vi "Verify Message Type.vi"(8 "error in":errorcluster, 11 "message type in":string) -> (0 "error out":errorcluster, 3 "message type out":T1, 4 "expected RT direction":string, 6 "number of expected addresses":i32)   [LabVIEW 2020, in "MIL-STD 1553 Import.lvlib"]
uses:
  MIL-STD 1553 Import.lvlib
  Shared/Message Type.ctl
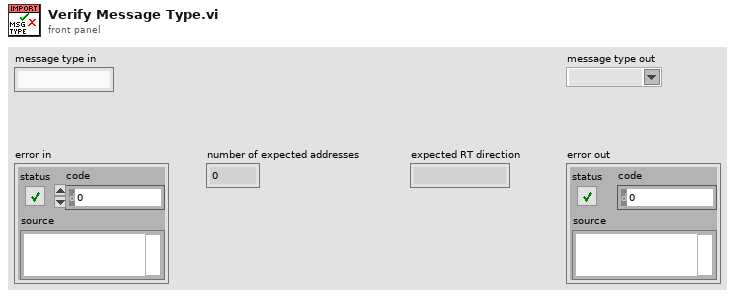
[diagram p1: front panel]
types:
  T1 = typedef "Message Type.ctl" = string
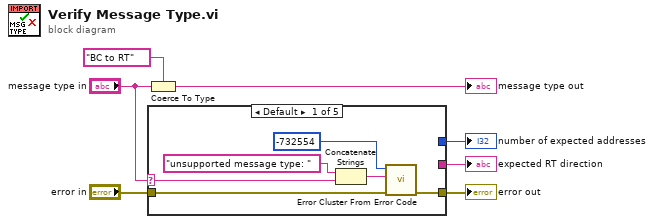
[diagram p0: block diagram]
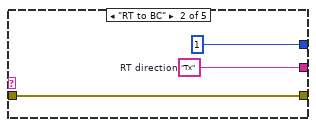
[diagram p2: hidden frame]
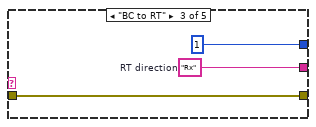
[diagram p3: hidden frame]
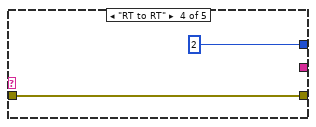
[diagram p4: hidden frame]
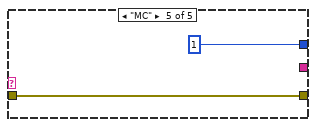
[diagram p5: hidden frame]
diagram:
  n1 = Coerce To Type(0:"message type in", 1:T1 "BC to RT" ("message type")) -> (2:→"message type out":T1)
  n2 = case shown="Default" "message type in" {
    selector: "message type in" -> [w10 _ _ _ _]
    tunnel: [w12 w16 w19 w21 w23] -> w7
    tunnel: "error in" -> [w13 w16 w19 w21 w23]
    tunnel: [_ 1 1 2 1] -> w4
    tunnel: [_ w14 w17 _ _] -> w3
    frame Default {
      n3 = Concatenate Strings("unsupported message type: ", w10) -> (w9:string)
      n4 = call <vilib>:"Error Cluster From Error Code.vi"("error in (no error)"=w13, "error message (\"\")"=w9, "error code (0)"=-732554) -> ("error out"=w12:errorcluster)  [unwired: 6 in]
    }
    frame "RT to BC" {
      w14 = "Tx"  # RT direction
    }
    frame "BC to RT" {
      w17 = "Rx"  # RT direction
    }
    frame "RT to RT" {
    }
    frame "MC" {
    }
  }
  "number of expected addresses" <- w4
  "expected RT direction" <- w3
  "error out" <- w7
